vi "AssertTrueOrFalse_Tests.vi"(11 "error in (no error)":errorcluster) -> (15 "error out":errorcluster)   [LabVIEW 2016, in "DronaTest.lvlib"]
uses:
  DronaTest.lvlib
  APIs/Assert/AssertControlValue/False.vi
  <vilib>/addons/_JKI Toolkits/Caraya/classes/Assert/Assert Error.vi
  APIs/Assert/AssertControlValue/True.vi
  <vilib>/addons/_JKI Toolkits/Caraya/classes/Assert/Assert Equal Value_Variant.vi
  <vilib>/addons/_JKI Toolkits/Caraya/classes/Test/Test.lvclass
  Drona.lvlib
  <vilib>/addons/_JKI Toolkits/Caraya/classes/Assert/Assert.lvclass
  APIs/Assert/AssertControlValue/AssertControlValue.lvlib
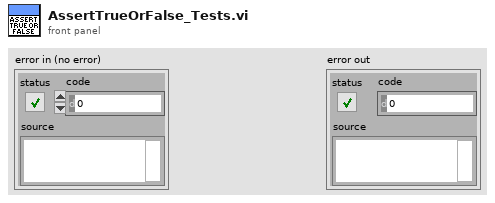
[diagram p1: front panel]
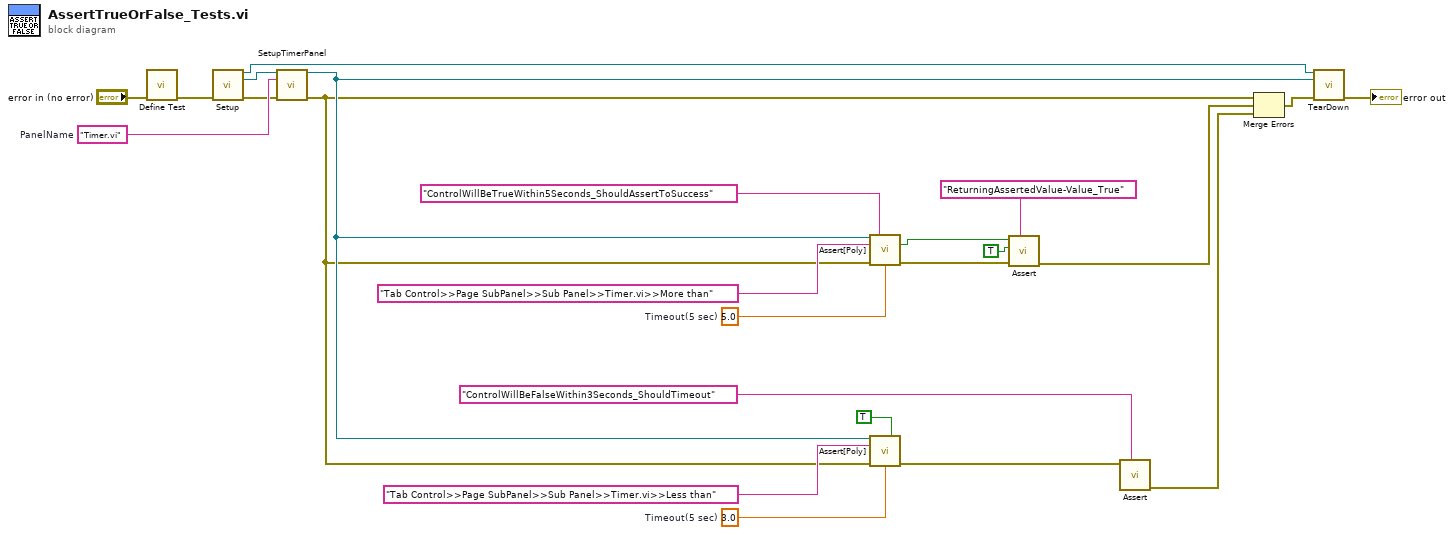
[diagram p0: block diagram]
diagram:
  w15 = "Timer.vi"  # PanelName
  w20 = 3.0  # Timeout(5 sec)
  w21 = 5.0  # Timeout(5 sec)
  n1 = call <vilib>:"Define Test.vi"("error in (no error)"="error in (no error)") -> ("error out"=w12:errorcluster)  [unwired: 9 in, 1 out]
  n2 = call "Setup.vi"("error in (no error)"=w12) -> ("Application Ref"=w8:refnum<vi>, "VI out"=w13:refnum<vi>, "error out"=w14:errorcluster)  [unwired: 12 in]
  n3 = call "SetupTimerPanel.vi"("VI in"=w13, "Panel Name"=w15, "error in (no error)"=w14) -> ("VI out"=w11:refnum<vi>, "error out"=w7:errorcluster)  [unwired: 11 in]
  n4 = call-poly "Assert[Poly].vi"("VI Reference In"=w11, "Test Label"="ControlWillBeTrueWithin5Seconds_ShouldAssertToSuccess" ("string"), "Control Path"="Tab Control>>Page SubPanel>>Sub Panel>>Timer.vi>>More than", "Error In"=w7, "Timeout(5 sec)"=w21) -> ("Asserted Value"=w4:bool, "Error Out"=w6:errorcluster)  [unwired: 8 in, 1 out]
  n5 = call-poly "Assert[Poly].vi"("VI Reference In"=w11, "Assert Only? (F)"=TRUE, "Control Path"="Tab Control>>Page SubPanel>>Sub Panel>>Timer.vi>>Less than", "Error In"=w7, "Timeout(5 sec)"=w20) -> ("Error Out"=w2:errorcluster)  [unwired: 8 in, 2 out]
  n6 = call-poly <vilib>:"Assert.vi"("Label"="ReturningAssertedValue-Value_True", "error in (no error)"=w6, "Y"=TRUE ("Asserted Value"), "X"=w4) -> ("error out"=w5:errorcluster)  [unwired: 6 in, 1 out]
  n7 = call-poly <vilib>:"Assert.vi"("Label"="ControlWillBeFalseWithin3Seconds_ShouldTimeout" ("string"), "Error?"=w2) -> ("error out"=w16:errorcluster)  [unwired: 8 in, 1 out]
  n8 = Merge Errors(w7, w5, w16) -> (w10:errorcluster)
  n9 = call "TearDown.vi"("Application Ref"=w8, "VI in"=w11, "error in (no error)"=w10) -> ("error out"=→"error out":errorcluster)  [unwired: 12 in]
